vi "Get Camera Object.vi"() -> (0 "error out":errorcluster, 3 "Camera out":refnum<class "Camera.lvclass">)   [LabVIEW 2016, in "Camera.lvclass"]
uses:
  Camera.lvclass
  Copy of Edmund Optics Folder/Edmund Optics.lvclass
  D:/INTT/Classes/Controllers/Camera/Copy of Camera Folder/Camera.lvclass
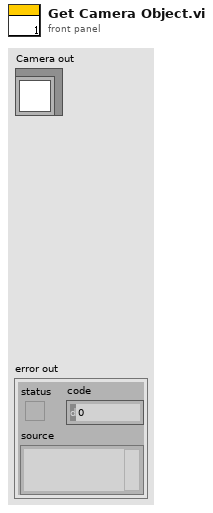
[diagram p1: front panel]
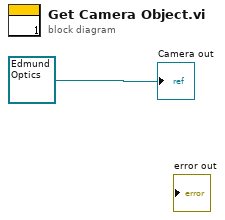
[diagram p0: block diagram]
diagram:
  "Camera out" <- refnum<class "Edmund Optics.lvclass"> refnum ("Copy of Edmund Optics.lvclass")
